vi "Write and Read.vi"(6 "Num bytes":u32=1024, 7 "Timeout (ms)":u32=10000, 8 "Error in (no error)":errorcluster, 10 "Command":string="*IDN?", 11 "VISA resource":refnum<visa-resource-name>) -> (0 "Error out":errorcluster, 1 "Error description":string, 2 "Response":string, 3 "Dup VISA resource":refnum<visa-resource-name>, 4 "Status Bytes":u16[](array[numeric]))   [LabVIEW 2010]
doc: "Copyright (c) 2012 Metrolab Technology SA, Plan-les-Ouates, Geneva, Switzerland\nWrite a command to the instrument and read the response.\nNearly all the commands issued by the instrument API pass through this VI.\nIt is highly recommended that any custom commands also use this utility VI."
panel:
  # "Write & Read"
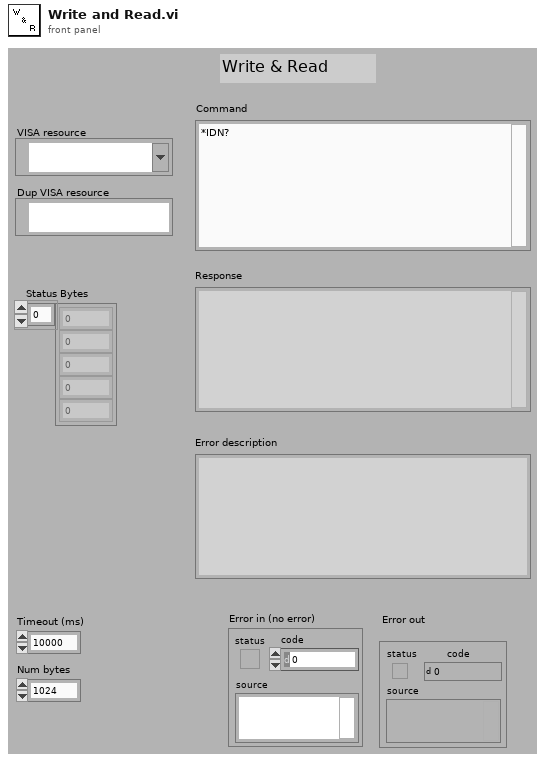
[diagram p1: front panel]
types:
  T1 = typedef "Semaphore RefNum" = refnum<k1>
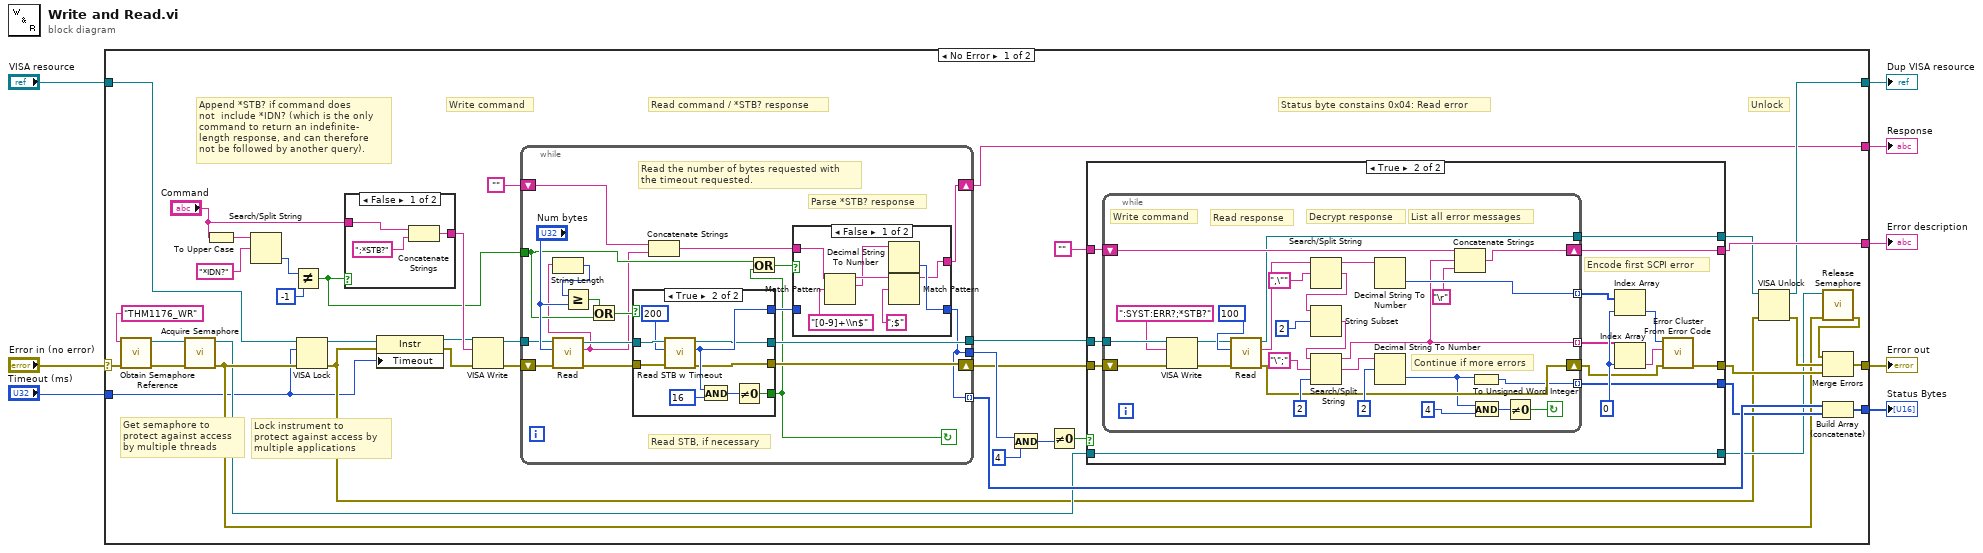
[diagram p0: block diagram]
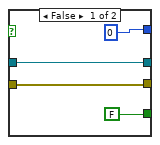
[diagram p4: hidden frame]
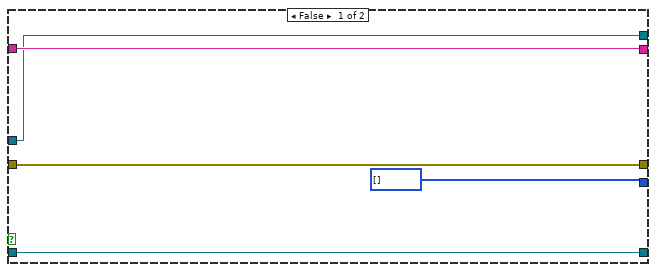
[diagram p5: hidden frame]
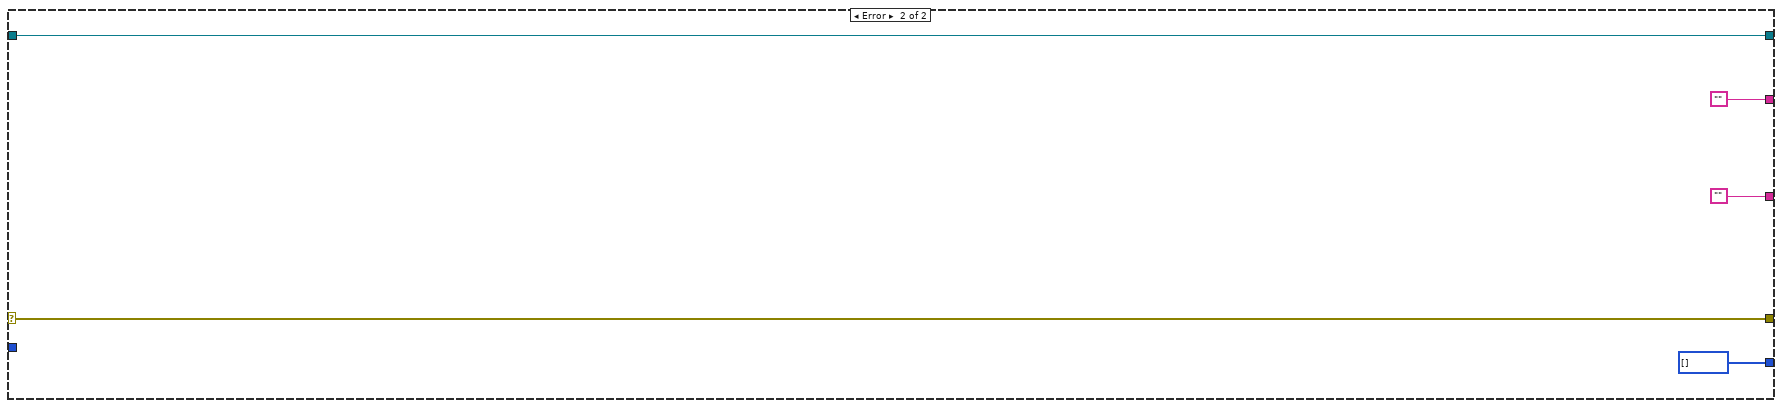
[diagram p6: hidden frame]
diagram:
  n1 = case shown="No Error" "Error in (no error)" {
    selector: "Error in (no error)" -> [w32 w144]
    tunnel: [w28 w144] -> w8
    tunnel: [w49 "" ("read buffer")] -> w7
    tunnel: [w13 "" ("read buffer")] -> w6
    tunnel: [w47 u16[] []] -> w4
    tunnel: "VISA resource" -> [w33 w142]
    tunnel: [w34 w142] -> w2
    tunnel: "Timeout (ms)" -> [w16 _]
    frame No Error {
      # "Get semaphore to\nprotect against access\nby multiple threads"
      # "Unlock"
      # "Lock instrument to\nprotect against access by\nmultiple applications"
      # "Status byte constains 0x04: Read error"
      # "Append *STB? if command does\nnot  include *IDN? (which is the only\ncommand to return an indefinite-\nlength response, and can therefore\nnot be followed by another query)."
      # "Read command / *STB? response"
      # "Write command"
      n2 = call <vilib>:"Obtain Semaphore Reference.vi"("error in (no error)"=w32, "name (unnamed)"="THM1176_WR") -> ("error out"=w31:errorcluster, "semaphore"=w29:T1)  [unwired: 3 in, 1 out]
      n3 = call <vilib>:"Acquire Semaphore.vi"("error in (no error)"=w31, "semaphore"=w29) -> ("error out"=w24:errorcluster, "semaphore out"=w23:T1)  [unwired: 3 in, 1 out]
      n4 = To Upper Case(1:"Command") -> (0:w10:string)
      n5 = Search/Split String(string=w10, search string/char (-)="*IDN?" ("y")) -> (offset of match=w15:i32)  [unwired: 1 in, 2 out]
      n6 = Not Equal?(x=w15, y=-1) -> (x != y?=w21:bool)
      n7 = VISA Lock(8:w24, 10:w16, 11:w33) -> (0:w19:errorcluster, 3:w20:refnum<visa-resource-name>)  [unwired: 2 in, 1 out]
      n8 = case shown="False" w21 {
        tunnel: "Command" -> [w51 w53]
        tunnel: [w50 w53] -> w40
        frame False {
          n9 = Concatenate Strings(w51, ";*STB?") -> (w50:string)
        }
        frame True {
        }
      }
      n10 = property class="Instr"(reference=w20, error in=w19, "Timeout"=w16) -> (reference out=w18:refnum<visa-resource-name>, error out=w17:errorcluster)
      n11 = VISA Write(VISA resource name=w18, write buffer=w40, error in (no error)=w17) -> (VISA resource name out=w39:refnum<visa-resource-name>, error out=w41:errorcluster)  [unwired: 1 out]
      n12 = while {
        shift-right: [w55] -> w13
        shift-left: "" ("read buffer") -> [w72]
        tunnel: [w62] -> w12
        shift-right: [w63] -> w11
        shift-left: w41 -> [w66]
        tunnel: [w54] -> w42
        tunnel: w39 -> [w67]
        tunnel: [w54] -> w48 mode=indexing
        tunnel: w21 -> [w60]
        stop <- w59 continue-if-true
        # "Parse *STB? response"
        # "Read STB, if necessary"
        # "Read the number of bytes requested with\nthe timeout requested."
        n13 = call "Read.vi"("Error in (no error)"=w66, "Byte count"="Num bytes", "VISA resource"=w67) -> ("Error out"=w64:errorcluster, "Read buffer"=w57:string, "Dup VISA resource"=w65:refnum<visa-resource-name>)  [unwired: 5 in, 1 out]
        n14 = String Length(string=w57) -> (length=w71:i32)
        n15 = Greater Or Equal?(x=w71, y="Num bytes") -> (x >= y?=w69:bool)
        n16 = Or(x=w69, y=w60) -> (x .or. y?=w68:bool)
        n17 = case shown="True" w68 {
          tunnel: [FALSE w92] -> w59
          tunnel: [u16 0 ("status byte") w91] -> w61
          tunnel: w65 -> [w83 w90]
          tunnel: [w83 w89] -> w62
          tunnel: w64 -> [w84 w88]
          tunnel: [w84 w87] -> w63
          frame False {
          }
          frame True {
            n18 = call "Read STB w Timeout.vi"("error in (no error)"=w88, "STB timeout"=u32 200, "VISA resource name"=w90) -> ("error out"=w87:errorcluster, "status byte"=w91:u16, "VISA resource name out"=w89:refnum<visa-resource-name>)  [unwired: 6 in]
            n19 = And(x=w91, y=u16 16) -> (x .and. y?=w93:u16)
            n20 = Not Equal To 0?(x=w93) -> (x != 0?=w92:bool)
          }
        }
        n21 = Concatenate Strings(w72, w57) -> (w56:string)
        n22 = Or(x=w60, y=w59) -> (x .or. y?=w58:bool)
        n23 = case shown="False" w58 {
          tunnel: w56 -> [w78 w81]
          tunnel: [w73 w81] -> w55
          tunnel: w61 -> [_ w80]
          tunnel: [w74 w80] -> w54
          frame False {
            n24 = Match Pattern(string=w78, regular expression="[0-9]+\\n$") -> (before substring=w77:string, match substring=w75:string)  [unwired: 1 in, 2 out]
            n25 = Decimal String To Number(string=w75) -> (number=w74:i32)  [unwired: 2 in, 1 out]
            n26 = Match Pattern(string=w77, regular expression=";$") -> (before substring=w73:string)  [unwired: 1 in, 3 out]
          }
          frame True {
          }
        }
      }
      n27 = And(x=w42, y=u16 4) -> (x .and. y?=w46:i32)
      n28 = Not Equal To 0?(x=w46) -> (x != 0?=w45:bool)
      n29 = case shown="True" w45 {
        tunnel: w12 -> [w97 w113]
        tunnel: w11 -> [w99 w110]
        tunnel: [w99 w107] -> w25
        tunnel: "" ("read buffer") -> [w98 w112]
        tunnel: [w98 w111] -> w49
        tunnel: [u16[] [] w102] -> w37
        tunnel: [w97 w101] -> w35
        tunnel: w23 -> [w95 w100]
        tunnel: [w95 w100] -> w22
        frame False {
        }
        frame True {
          w109 = 0 ("index")
          # "Encode first SCPI error"
          n30 = while {
            tunnel: w113 -> [w141]
            shift-right: [w138] -> w111
            shift-left: w112 -> [w137]
            shift-right: [w124] -> w108
            shift-left: w110 -> [w134]
            tunnel: [w123] -> w106 mode=indexing
            tunnel: [w126] -> w103 mode=indexing
            tunnel: [w115] -> w102 mode=indexing
            tunnel: [w114] -> w101
            stop <- w139 continue-if-true
            # "Decrypt response"
            # "Read response"
            # "Write command"
            # "Continue if more errors"
            # "List all error messages"
            n31 = VISA Write(VISA resource name=w141, write buffer=":SYST:ERR?;*STB?" ("string to write 2"), error in (no error)=w134) -> (VISA resource name out=w133:refnum<visa-resource-name>, error out=w132:errorcluster)  [unwired: 1 out]
            n32 = call "Read.vi"("Error in (no error)"=w132, "Byte count"=u32 100 ("byte count"), "VISA resource"=w133) -> ("Error out"=w124:errorcluster, "Read buffer"=w129:string, "Dup VISA resource"=w114:refnum<visa-resource-name>)  [unwired: 5 in, 1 out]
            n33 = Search/Split String(string=w129, search string/char (-)=",\"") -> (substring before match=w127:string, match + rest of string=w121:string)  [unwired: 1 in, 1 out]
            n34 = String Subset(string=w121, offset (0)=2) -> (substring=w119:string)  [unwired: 1 in]
            n35 = Search/Split String(string=w119, search string/char (-)="\";", offset (0)=2) -> (substring before match=w123:string, match + rest of string=w117:string)  [unwired: 1 out]
            n36 = Decimal String To Number(string=w127) -> (number=w126:i32)  [unwired: 2 in, 1 out]
            n37 = Decimal String To Number(string=w117, offset=2) -> (number=w116:i32)  [unwired: 1 in, 1 out]
            n38 = Concatenate Strings(w137, w123, "\r") -> (w138:string)
            n39 = To Unsigned Word Integer(number=w116) -> (unsigned 16bit integer=w115:u16)
            n40 = And(x=w116, y=4) -> (x .and. y?=w140:i32)
            n41 = Not Equal To 0?(x=w140) -> (x != 0?=w139:bool)
          }
          n42 = Index Array(array=w103, index=w109) -> (element=w104:i32)
          n43 = Index Array(array=w106, index=w109) -> (element=w105:string)
          n44 = call <vilib>:"Error Cluster From Error Code.vi"("error in (no error)"=w108, "error message (\"\")"=w105, "error code (0)"=w104) -> ("error out"=w107:errorcluster)  [unwired: 1 in, 5 out]
        }
      }
      n45 = VISA Unlock(8:w19, 11:w35) -> (0:w27:errorcluster, 3:w34:refnum<visa-resource-name>)
      n46 = call <vilib>:"Release Semaphore.vi"("error in (no error)"=w24, "semaphore"=w22) -> ("error out"=w26:errorcluster)  [unwired: 4 in, 1 out]
      n47 = Merge Errors(w26, w27, w25) -> (w28:errorcluster)
      n48 = Build Array (concatenate)(w48, w37) -> (w47:i32[])
    }
    frame Error {
    }
  }
  "Error out" <- w8
  "Error description" <- w7
  "Response" <- w6
  "Status Bytes" <- w4
  "Dup VISA resource" <- w2
